vi "FB_MFA_Set_Position1Enc0 -NxtMve.vi"(11 "Position Put":sgl) -> (2 "Position Get":sgl format="%.2f", 3 "SetPositionError":bool)   [LabVIEW 2011]
panel:
  out "error AAABuild":errorcluster
  out "error SetUSBlink":errorcluster
  out "AAABuild":i32
  in  "error in":errorcluster
  in  "MintController":refnum<k7>(container)
  out "error Position Get":errorcluster
  out "error Position Put":errorcluster
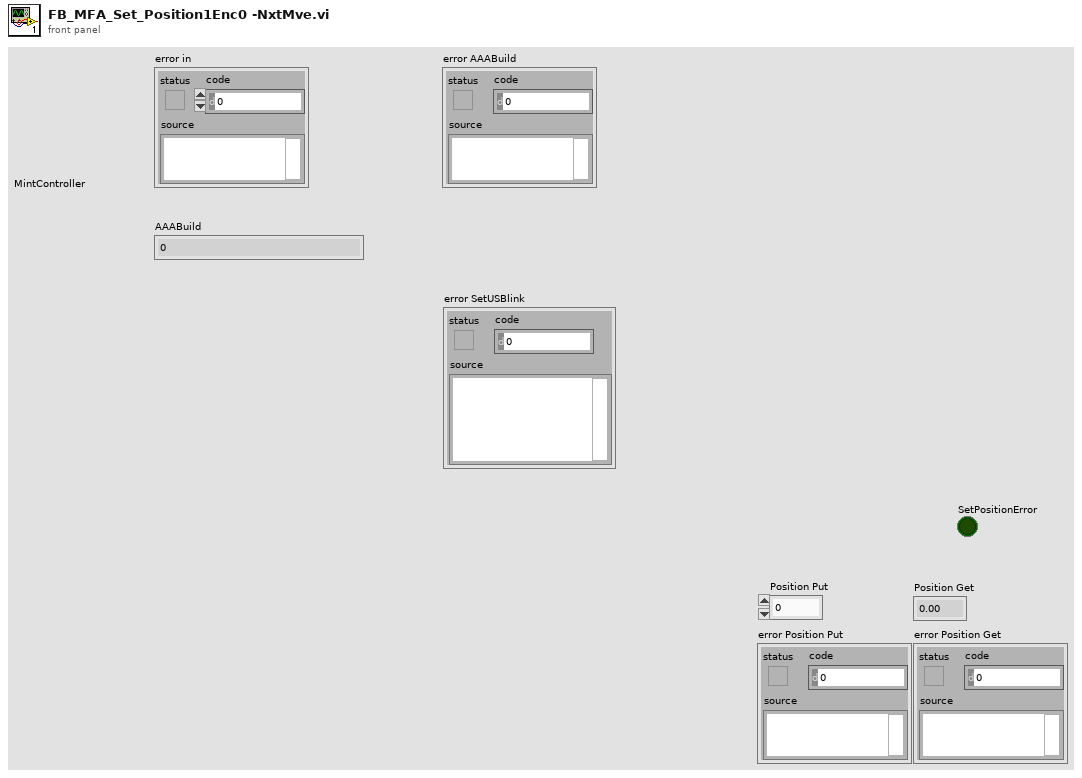
[diagram p1: front panel]
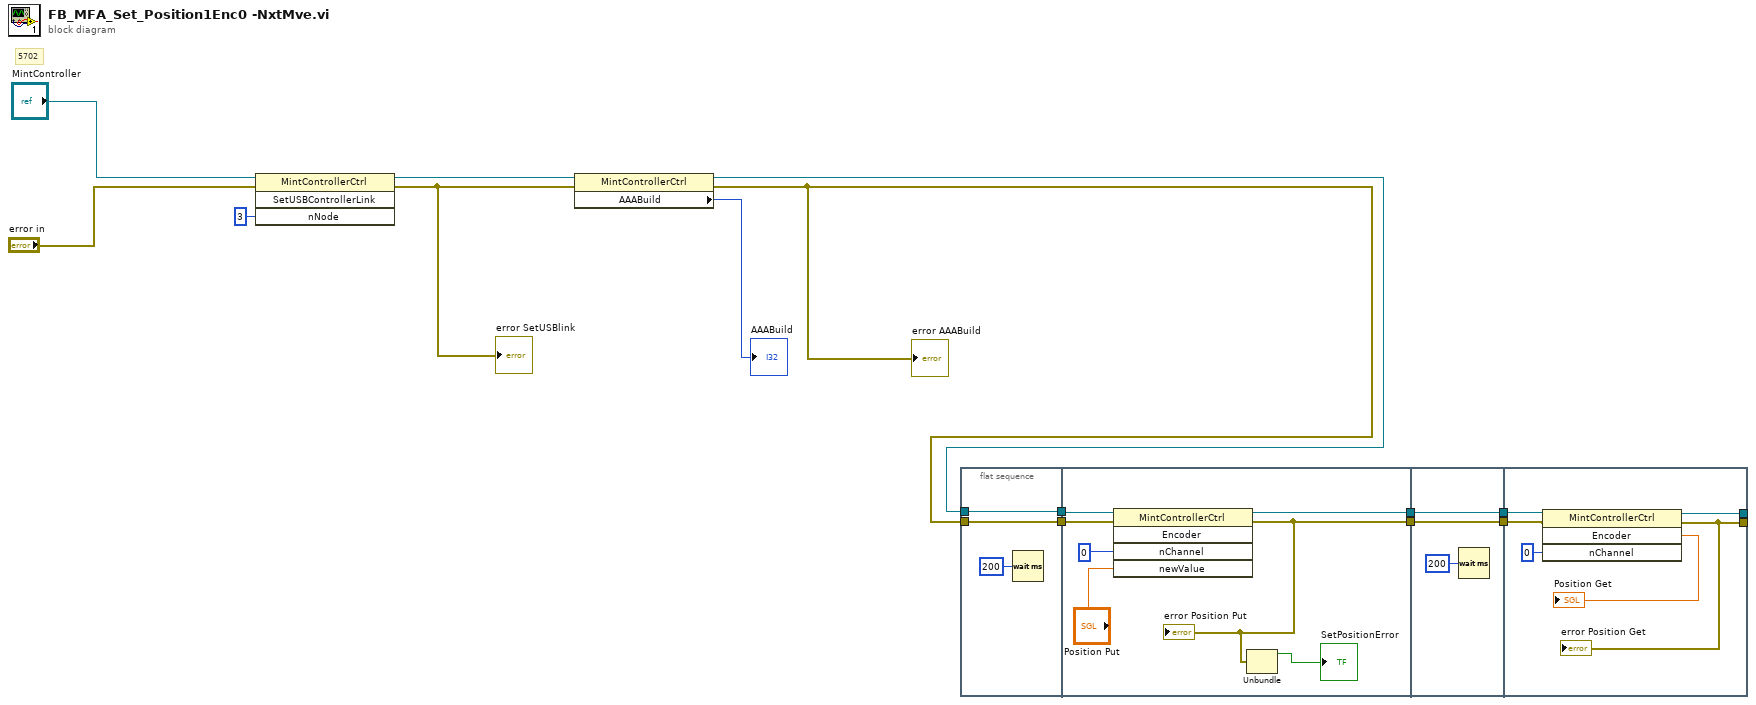
[diagram p0: block diagram]
diagram:
  # "5702"
  n1 = invoke class="MintControllerCtrl" method="SetUSBControllerLink"(reference="MintController", error in="error in", "nNode"=i16 3) -> (reference out=w4:refnum<k7>, error out=w3:errorcluster)  [unwired: 1 in, 2 out]
  "error SetUSBlink" <- w3
  n2 = property class="MintControllerCtrl"(reference=w4, error in=w3) -> (reference out=w2:refnum<k7>, error out=w1:errorcluster, "AAABuild"=→"AAABuild":i32)
  "error AAABuild" <- w1
  n3 = flat-sequence {
    tunnel: [w17] -> w14
    tunnel: [w16] -> w13
    tunnel: w1 -> [w17]
    tunnel: w2 -> [w16]
    tunnel: w14 -> [w23]
    tunnel: w13 -> [w22]
    tunnel: [w21] -> w12
    tunnel: [w19] -> w11
    tunnel: w12 -> [w27]
    tunnel: w11 -> [w26]
    tunnel: [w27] -> w10
    tunnel: [w26] -> w9
    tunnel: w10 -> [w33]
    tunnel: w9 -> [w32]
    tunnel: [w29] -> _
    tunnel: [w28] -> _
    frame #0 {
      n4 = Wait (ms)(milliseconds to wait=u32 200) -> ()  [unwired: 1 out]
    }
    frame #1 {
      n5 = invoke class="MintControllerCtrl" method="Encoder"(reference=w22, error in=w23, "nChannel"=i16 0 ("nAxis"), "newValue"="Position Put") -> (reference out=w21:refnum<k7>, error out=w19:errorcluster)  [unwired: 1 in, 3 out]
      "error Position Put" <- w19
      n6 = Unbundle(w19) -> ("status"=→"SetPositionError":bool)  [unwired: 2 out]
    }
    frame #2 {
      n7 = Wait (ms)(milliseconds to wait=u32 200) -> ()  [unwired: 1 out]
    }
    frame #3 {
      n8 = invoke class="MintControllerCtrl" method="Encoder"(reference=w33, error in=w32, "nChannel"=i16 0 ("nBank")) -> (reference out=w29:refnum<k7>, error out=w28:errorcluster, "Encoder"=→"Position Get":sgl)  [unwired: 1 in, 1 out]
      "error Position Get" <- w28
    }
  }
